vi "New PI_1.vi"(0 "CtrlIndex":i32, 1 "LimitsArray":cluster{"Step":dbl, "Max":dbl, "Min":dbl}[](array[cluster]), 2 "FFinfo":T1(array[cluster]), 3 "PIinfo":T2(array[cluster]), 5 "CommandCluster":T4, 6 "Run?":bool, 7 "Feedback":dbl[](array[numeric]), 9 "CutoffArray":cluster{"MidCutoff":dbl, "CloseCutoff":dbl}[](array[cluster]), 11 "Stability In":T3, 12 "Tolerances":dbl[](array[numeric]), 13 "Controller?":bool, 14 "Ave Feedback":dbl[](array[numeric])) -> (4 "PIdata":dbl[](array[numeric]), 8 "Output":dbl, 10 "Stable?":bool, 15 "Stability Out":T3)   [LabVIEW 2013]
uses:
  TypeDef/Command Cluster.ctl
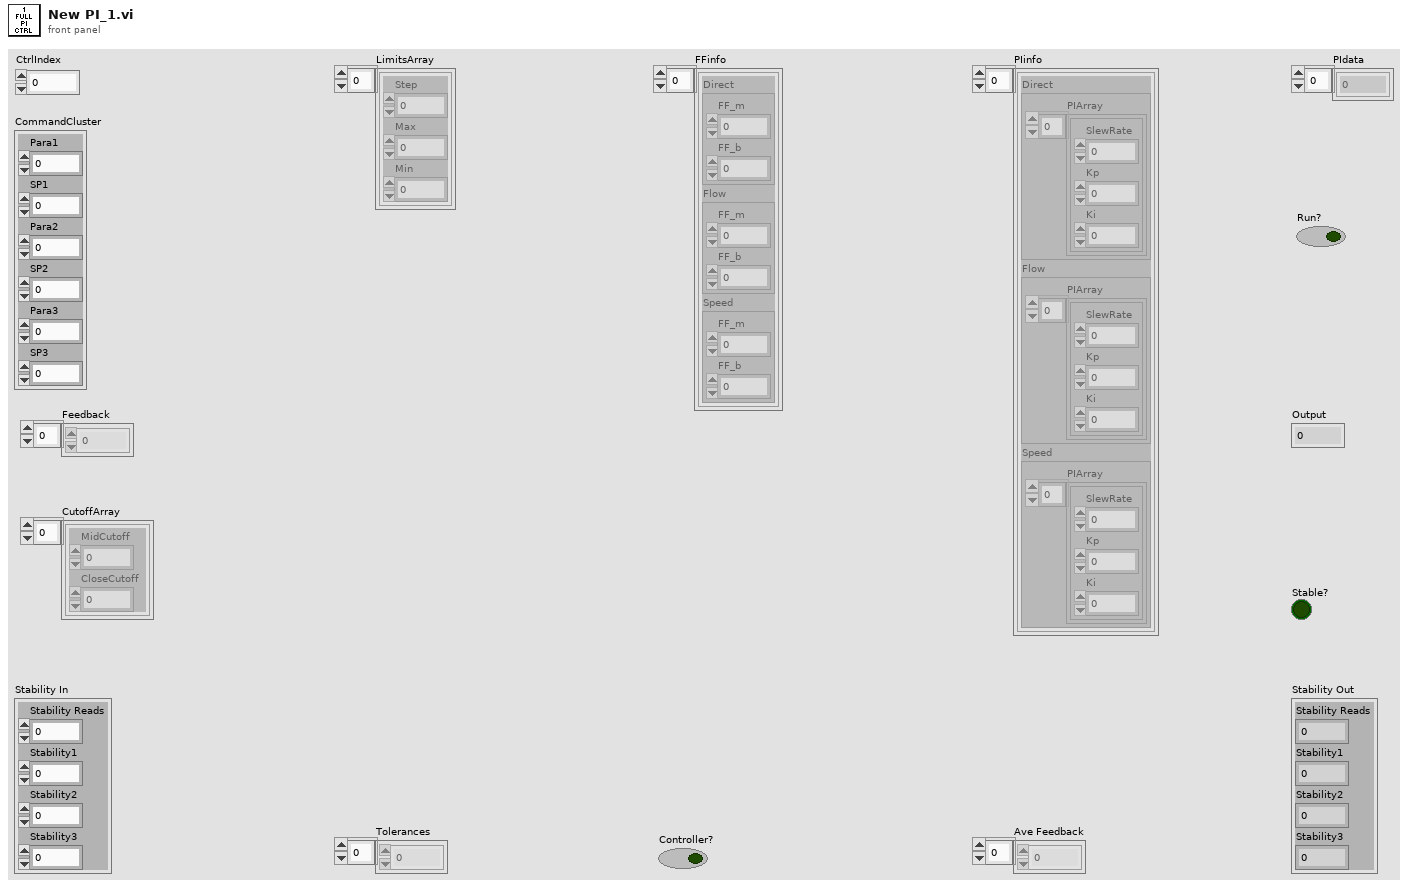
[diagram p1: front panel]
types:
  T1 = cluster{"Direct":cluster{"FF_m":dbl, "FF_b":dbl}, "Flow":cluster{"FF_m":dbl, "FF_b":dbl}, "Speed":cluster{"FF_m":dbl, "FF_b":dbl}}[]
  T2 = cluster{"Direct":cluster{"PIArray":cluster{"SlewRate":dbl, "Kp":dbl, "Ki":dbl}[]}, "Flow":cluster{"PIArray":cluster{"SlewRate":dbl, "Kp":dbl, "Ki":dbl}[]}, "Speed":cluster{"PIArray":cluster{"SlewRate":dbl, "Kp":dbl, "Ki":dbl}[]}}[]
  T3 = cluster{"Stability Reads":i32, "Stability1":i32, "Stability2":i32, "Stability3":i32}
  T4 = typedef "Command Cluster.ctl" = cluster{"Para1":i32, "SP1":dbl, "Para2":i32, "SP2":dbl, "Para3":i32, "SP3":dbl}
  T5 = cluster{"Direct":cluster{"FF_m":dbl, "FF_b":dbl}, "Flow":cluster{"FF_m":dbl, "FF_b":dbl}, "Speed":cluster{"FF_m":dbl, "FF_b":dbl}}
  T6 = cluster{"Direct":cluster{"PIArray":cluster{"SlewRate":dbl, "Kp":dbl, "Ki":dbl}[]}, "Flow":cluster{"PIArray":cluster{"SlewRate":dbl, "Kp":dbl, "Ki":dbl}[]}, "Speed":cluster{"PIArray":cluster{"SlewRate":dbl, "Kp":dbl, "Ki":dbl}[]}}
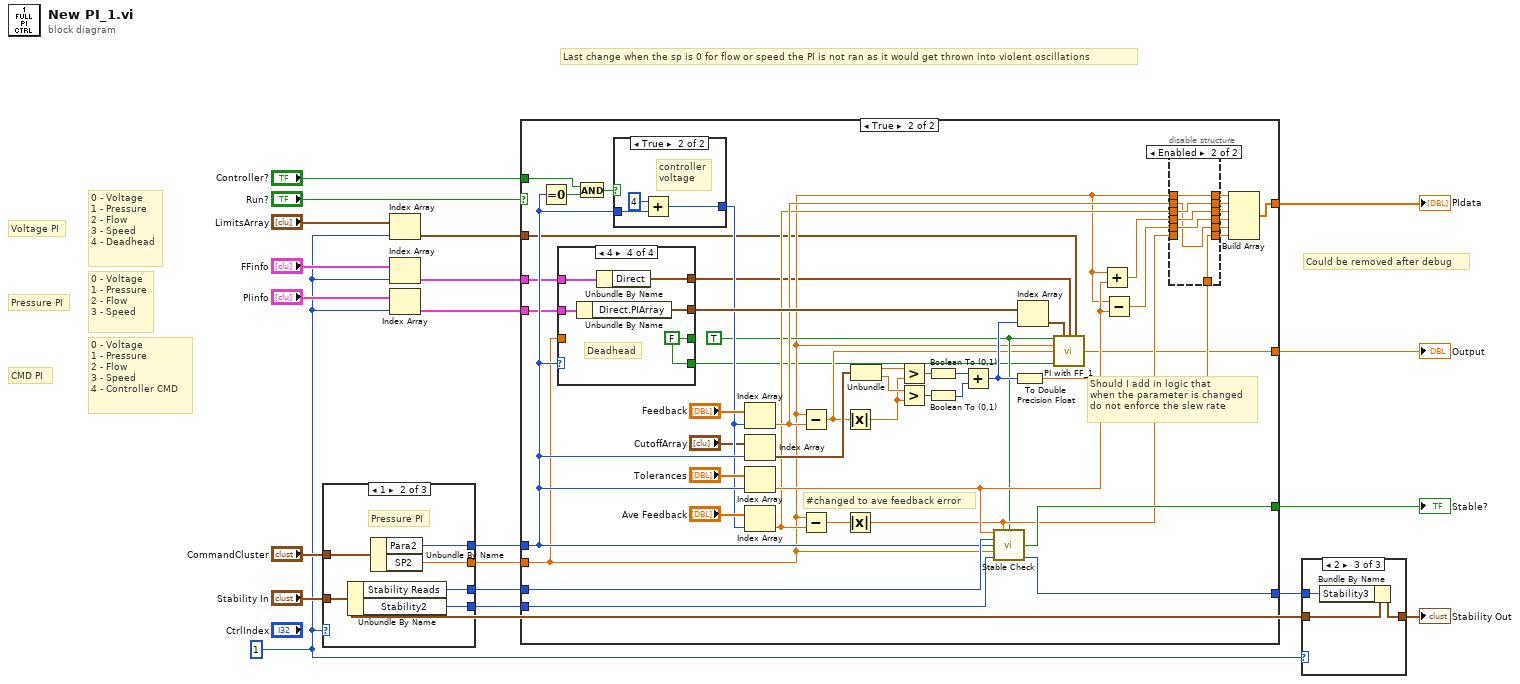
[diagram p0: block diagram]
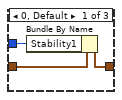
[diagram p2: hidden frame]
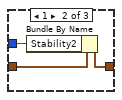
[diagram p3: hidden frame]
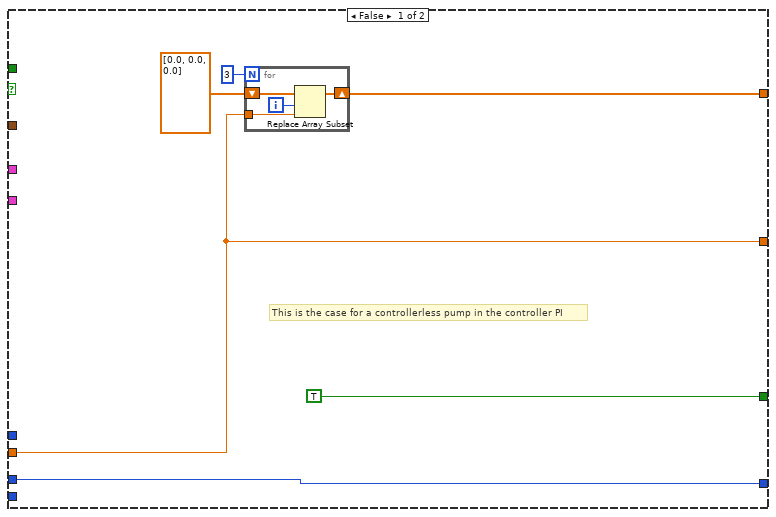
[diagram p4: hidden frame]
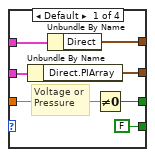
[diagram p7: hidden frame]
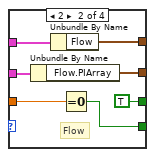
[diagram p8: hidden frame]
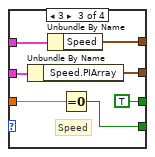
[diagram p9: hidden frame]
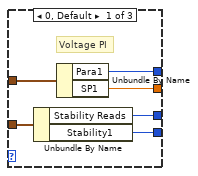
[diagram p10: hidden frame]
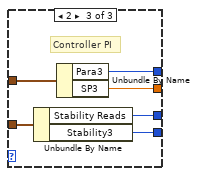
[diagram p11: hidden frame]
diagram:
  w2 = 1 ("CtrlIndex")
  # "Last change when the sp is 0 for flow or speed the PI is not ran as it would get thrown into violent oscillations"
  # "Could be removed after debug"
  # "CMD PI"
  # "Pressure PI"
  # "Voltage PI"
  # "0 - Voltage\n1 - Pressure\n2 - Flow\n3 - Speed\n4 - Controller CMD"
  # "0 - Voltage\n1 - Pressure\n2 - Flow\n3 - Speed"
  # "0 - Voltage\n1 - Pressure\n2 - Flow\n3 - Speed\n4 - Deadhead"
  n1 = case shown="1" w2 {
    tunnel: "Stability In" -> [w26 w32 w38]
    tunnel: [w24 w30 w36] -> w19
    tunnel: [w25 w31 w37] -> w18
    tunnel: "CommandCluster" -> [w23 w29 w35]
    tunnel: [w22 w28 w34] -> w17
    tunnel: [w21 w27 w33] -> w16
    frame 0, Default {
      # "Voltage PI"
      n2 = Unbundle By Name(w26) -> ("Stability Reads"=w24:i32, "Stability1"=w25:i32)
      n3 = Unbundle By Name(w23) -> ("Para1"=w22:i32, "SP1"=w21:dbl)
    }
    frame 1 {
      # "Pressure PI"
      n4 = Unbundle By Name(w32) -> ("Stability Reads"=w30:i32, "Stability2"=w31:i32)
      n5 = Unbundle By Name(w29) -> ("Para2"=w28:i32, "SP2"=w27:dbl)
    }
    frame 2 {
      # "Controller PI"
      n6 = Unbundle By Name(w38) -> ("Stability Reads"=w36:i32, "Stability3"=w37:i32)
      n7 = Unbundle By Name(w35) -> ("Para3"=w34:i32, "SP3"=w33:dbl)
    }
  }
  n8 = Index Array(array="LimitsArray", index=w2) -> (element=w7:cluster{"Step":dbl, "Max":dbl, "Min":dbl})
  n9 = Index Array(array="FFinfo", index=w2) -> (element=w3:T5)
  n10 = Index Array(array="PIinfo", index=w2) -> (element=w5:T6)
  n11 = case shown="True" "Run?" {
    tunnel: w19 -> [w43 w83]
    tunnel: w18 -> [_ w82]
    tunnel: w17 -> [_ w81]
    tunnel: w16 -> [w42 w55]
    tunnel: "Controller?" -> [_ w92]
    tunnel: [TRUE w71] -> w13
    tunnel: [w42 w49] -> w12
    tunnel: [w40 w91] -> w11
    tunnel: [w43 w84] -> w10
    tunnel: w7 -> [_ w50]
    tunnel: w5 -> [_ w79]
    tunnel: w3 -> [_ w77]
    frame False {
      # "This is the case for a controllerless pump in the controller PI"
      n12 = for {
        N: 3 -> [_]
        shift-right: [w47] -> w40
        shift-left: dbl[] [0.0, 0.0, 0.0] -> [w48]
        tunnel: w42 -> [w45]
        i -> [w46]
        n13 = Replace Array Subset(array=w48, new element=w45, index=w46) -> (w47:dbl[])
      }
    }
    frame True {
      w56 = TRUE
      # "#changed to ave feedback error"
      # "Should I add in logic that\nwhen the parameter is changed\ndo not enforce the slew rate"
      n14 = Equal To 0?(x=w81) -> (x = 0?=w95:bool)
      n15 = case shown="4" w81 {
        tunnel: [w113 TRUE TRUE w134] -> _
        tunnel: w79 -> [w119 w126 w133 w138]
        tunnel: [w118 w125 w132 w137] -> w78
        tunnel: w77 -> [w117 w124 w131 w136]
        tunnel: [w116 w123 w130 w135] -> w51
        tunnel: w55 -> [w114 w122 w129 _]
        tunnel: [FALSE w121 w128 w134] -> w53
        frame Default {
          # "Voltage or\nPressure"
          n16 = Unbundle By Name(w119) -> ("Direct.PIArray"=w118:cluster{"SlewRate":dbl, "Kp":dbl, "Ki":dbl}[])
          n17 = Unbundle By Name(w117) -> ("Direct"=w116:cluster{"FF_m":dbl, "FF_b":dbl})
          n18 = Not Equal To 0?(x=w114) -> (x != 0?=w113:bool)
        }
        frame 2 {
          # "Flow"
          n19 = Unbundle By Name(w126) -> ("Flow.PIArray"=w125:cluster{"SlewRate":dbl, "Kp":dbl, "Ki":dbl}[])
          n20 = Unbundle By Name(w124) -> ("Flow"=w123:cluster{"FF_m":dbl, "FF_b":dbl})
          n21 = Equal To 0?(x=w122) -> (x = 0?=w121:bool)
        }
        frame 3 {
          # "Speed"
          n22 = Unbundle By Name(w133) -> ("Speed.PIArray"=w132:cluster{"SlewRate":dbl, "Kp":dbl, "Ki":dbl}[])
          n23 = Unbundle By Name(w131) -> ("Speed"=w130:cluster{"FF_m":dbl, "FF_b":dbl})
          n24 = Equal To 0?(x=w129) -> (x = 0?=w128:bool)
        }
        frame 4 {
          w134 = FALSE
          # "Deadhead"
          n25 = Unbundle By Name(w138) -> ("Direct.PIArray"=w137:cluster{"SlewRate":dbl, "Kp":dbl, "Ki":dbl}[])
          n26 = Unbundle By Name(w136) -> ("Direct"=w135:cluster{"FF_m":dbl, "FF_b":dbl})
        }
      }
      n27 = And(x=w92, y=w95) -> (x .and. y?=w94:bool)
      n28 = case shown="True" w94 {
        tunnel: w81 -> [w109 w112]
        tunnel: [w109 w110] -> w75
        frame False {
          # "pump\nvoltage"
        }
        frame True {
          # "controller\nvoltage"
          n29 = Add(x=4, y=w112) -> (x+y=w110:i32)
        }
      }
      n30 = Index Array(array="Feedback", index=w75) -> (element=w69:dbl)
      n31 = Index Array(array="CutoffArray", index=w81) -> (element=w80:cluster{"MidCutoff":dbl, "CloseCutoff":dbl})
      n32 = Index Array(array="Tolerances", index=w81) -> (element=w70:dbl)
      n33 = Index Array(array="Ave Feedback", index=w75) -> (element=w68:dbl)
      n34 = Subtract(x=w55, y=w69) -> (x-y=w54:dbl)
      n35 = Subtract(x=w55, y=w68) -> (x-y=w74:dbl)
      n36 = Absolute Value(x=w54) -> (abs(x)=w73:dbl)
      n37 = Absolute Value(x=w74) -> (abs(x)=w65:dbl)
      n38 = Unbundle(w80) -> ("MidCutoff"=w86:dbl, "CloseCutoff"=w85:dbl)
      n39 = Greater?(x=w86, y=w73) -> (0:w90:bool)
      n40 = Greater?(x=w85, y=w73) -> (0:w89:bool)
      n41 = Boolean To (0,1)(Boolean=w90) -> (0, 1=w88:i16)
      n42 = Boolean To (0,1)(Boolean=w89) -> (0, 1=w87:i16)
      n43 = Add(x=w88, y=w87) -> (x+y=w59:i16)
      n44 = call "Stable Check.vi"("Tolerance"=w70, "AbsError"=w65, "PI Running?"=w56, "ReqReads"=w83, "Parameter"=w81, "Setpoint"=w55, "StabilityCount In"=w82) -> ("Stable?"=w71:bool, "StabilityCount Out"=w84:i32)  [unwired: 6 in, 1 out]
      n45 = To Double Precision Float(number=w59) -> (double precision float=w57:dbl)
      n46 = Index Array(array=w78, index=w59) -> (element=w52:cluster{"SlewRate":dbl, "Kp":dbl, "Ki":dbl})
      n47 = call "PI with FF_1.vi"("Run PI?"=w56, "PIcluster"=w52, "FFcluster"=w51, "LimitCluster"=w50, "SP"=w55, "Error"=w54, "RevCtrlZero"=w53) -> ("Output"=w49:dbl)  [unwired: 7 in, 1 out]
      n48 = Add(x=w55, y=w70) -> (x+y=w67:dbl)
      n49 = Subtract(x=w55, y=w70) -> (x-y=w66:dbl)
      n50 = disable-structure shown="Enabled" {
        disable-tunnel: w55 -> [w102 w108]
        disable-tunnel: w69 -> [w101 w104]
        disable-tunnel: w68 -> [w100 w107]
        disable-tunnel: w67 -> [w99 w106]
        disable-tunnel: w66 -> [w98 w105]
        disable-tunnel: w65 -> [w97 _]
        disable-tunnel: [w102 w108] -> w64
        disable-tunnel: [w101 w107] -> w63
        disable-tunnel: [w100 w106] -> w62
        disable-tunnel: [w99 w105] -> w61
        disable-tunnel: [w98 w104] -> w60
        disable-tunnel: [w97 w103] -> w58
        disable-tunnel: w57 -> [_ w103]
        frame Disabled {
        }
        frame Enabled {
        }
      }
      n51 = Build Array(w64, w63, w62, w61, w60, w58) -> (w91:dbl[])
    }
  }
  "Stable?" <- w13
  "Output" <- w12
  "PIdata" <- w11
  n52 = case shown="2" w2 {
    tunnel: "Stability In" -> [w140 w143 w146]
    tunnel: [w139 w142 w145] -> w14
    tunnel: w10 -> [w141 w144 w147]
    frame 0, Default {
      n53 = Bundle By Name(cluster=w140, "Stability1"=w141) -> (w139:T3)
    }
    frame 1 {
      n54 = Bundle By Name(cluster=w143, "Stability2"=w144) -> (w142:T3)
    }
    frame 2 {
      n55 = Bundle By Name(cluster=w146, "Stability3"=w147) -> (w145:T3)
    }
  }
  "Stability Out" <- w14
